vi "Rotate_Angle.vi"(7 "Direction of Rotation":T1, 8 "error in (no error)":errorcluster, 10 "Angle (degrees)":refnum<class "Angle.lvclass">, 11 "CartesianVector in":refnum<class "CartesianVector.lvclass">) -> (0 "error out":errorcluster, 3 "CartesianVector out":refnum<class "CartesianVector.lvclass">)   [LabVIEW 2012, in "CartesianVector.lvclass"]
doc: "Takes in a CartesianVector object, a direction of rotation, and an Angle object. Returns a new CartesianVector object that has been rotated by that angle either clockwise or counterclockwise."
uses:
  CartesianVector.lvclass
  Angles/Angle/Angle.lvclass
  TypeDefs/DirectionOfRotation.ctl
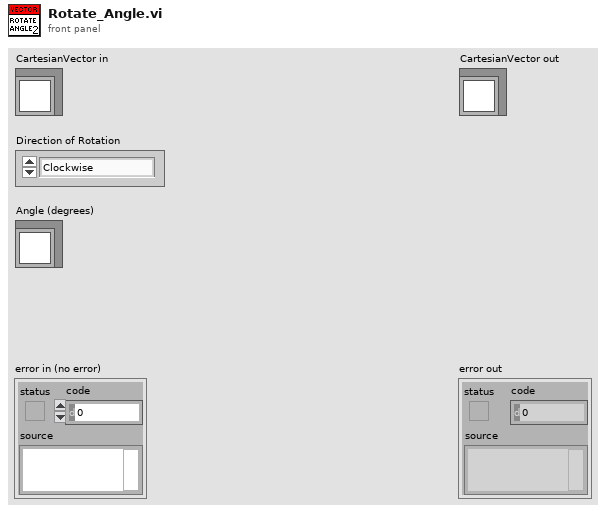
[diagram p1: front panel]
types:
  T1 = typedef "DirectionOfRotation.ctl" = enum16{"Clockwise", "Counter-Clockwise"}
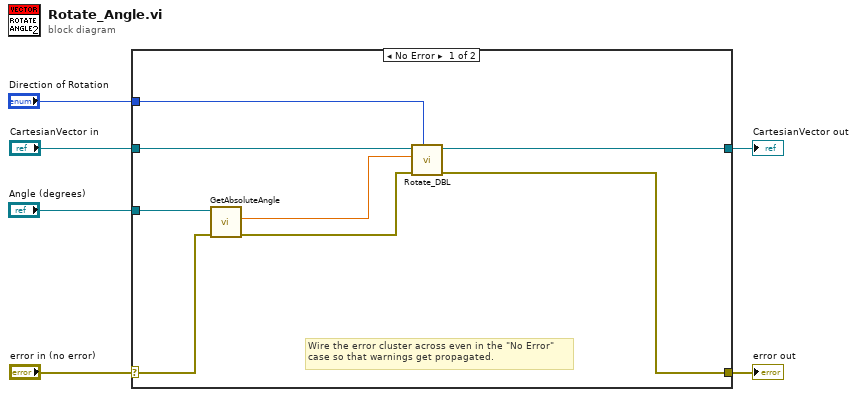
[diagram p0: block diagram]
diagram:
  n1 = case shown="No Error" "error in (no error)" {
    selector: "error in (no error)" -> [w12 w16]
    tunnel: [w9 w16] -> w5
    tunnel: [w8 w15] -> w3
    tunnel: "CartesianVector in" -> [w14 w15]
    tunnel: "Angle (degrees)" -> [w13 _]
    tunnel: "Direction of Rotation" -> [w7 _]
    frame No Error {
      # "Wire the error cluster across even in the \"No Error\"\ncase so that warnings get propagated."
      n2 = call "GetAbsoluteAngle.vi"("error in (no error)"=w12, "Angle in"=w13) -> ("error out"=w11:errorcluster, "Absolute angle (Deg.)"=w10:dbl)  [unwired: 8 in]
      n3 = call "Rotate_DBL.vi"("Direction of Rotation"=w7, "error in (no error)"=w11, "Angle (degrees)"=w10, "CartesianVector in"=w14) -> ("error out"=w9:errorcluster, "CartesianVector out"=w8:refnum<class "CartesianVector.lvclass">)  [unwired: 6 in]
    }
    frame Error {
    }
  }
  "error out" <- w5
  "CartesianVector out" <- w3
